vi "xeva-init.vi"() -> (0 "error out":errorcluster, 1 "initialized":bool, 2 "xeva-camref":T2)   [LabVIEW 2015]
uses:
  <vilib>/Xenics Infrared Solutions/Xeneth LabVIEW API/VIs/Controls/Camara.ctl
  <vilib>/Xenics Infrared Solutions/Xeneth LabVIEW API/Xeneth.lvlib
panel:
  in  "settings-file":path=path "D:/Programs/LabView/xenics-xeva-labview/settings/settings-integrationtime15s.xcf"
  in  "calibration-file":path=path "D:/Programs/LabView/xenics-xeva-labview/settings/calibration-170816-15000000us_2795.xca"
  in  "connection-type":T1(ring)=enum."automatic"
  out "status array":bool[](array[boolean])
  # "automatic mode"
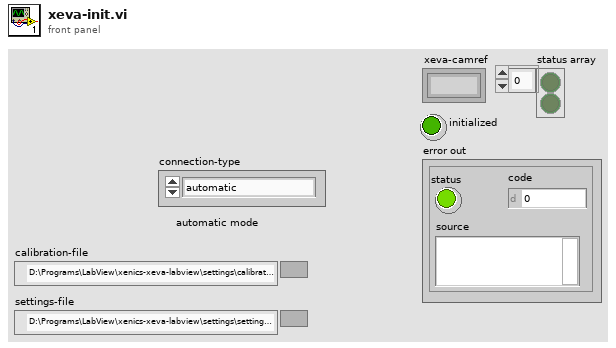
[diagram p1: front panel]
types:
  T1 = enum16{"interactive", "semi-interactive", "automatic"}
  T2 = typedef "Xeneth.lvlib/Camara.ctl" = refnum<k1>
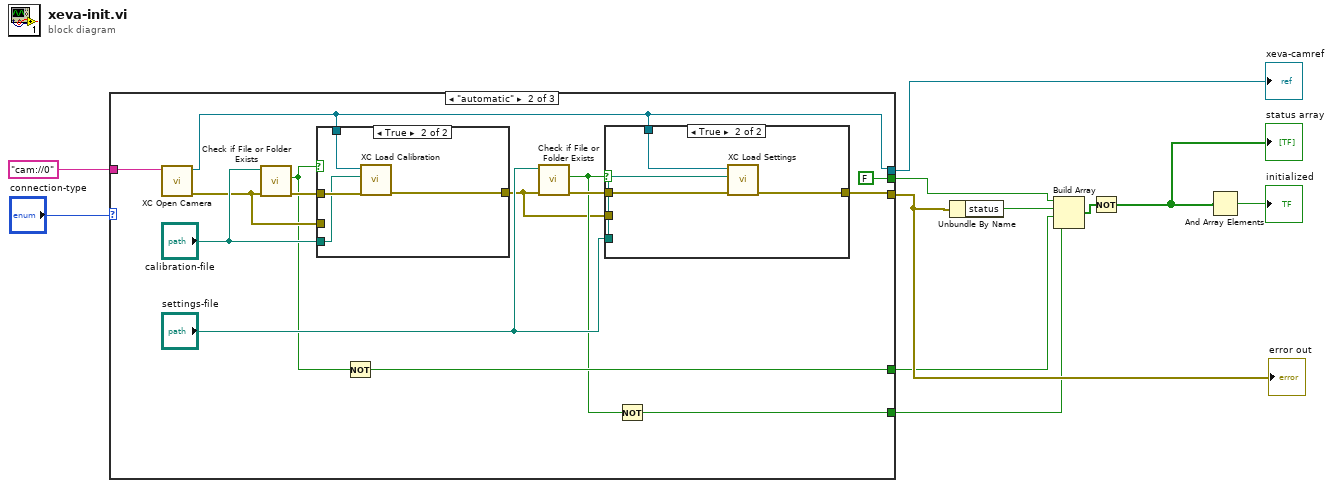
[diagram p0: block diagram]
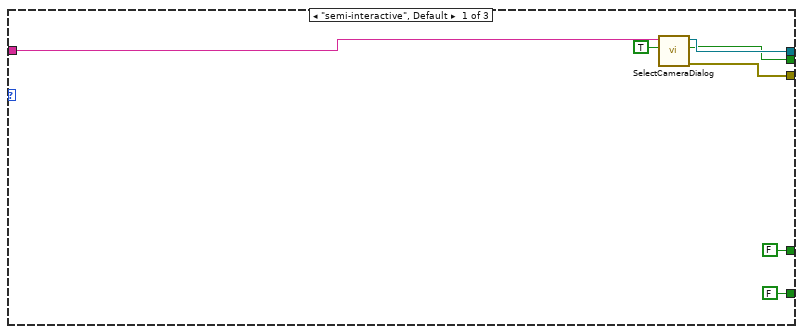
[diagram p2: hidden frame]
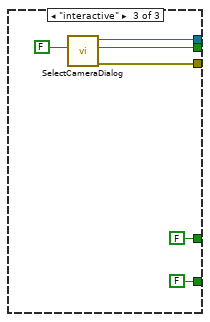
[diagram p5: hidden frame]
diagram:
  n1 = case shown="\"automatic\"" "connection-type" {
    tunnel: [w18 w19 w47] -> w11
    tunnel: [w16 w31 w46] -> w10
    tunnel: [w17 FALSE ("Cancelled") w45] -> w8
    tunnel: "cam://0" ("pCameraName") -> [w15 w32 _]
    tunnel: [FALSE w23 FALSE] -> w2
    tunnel: [FALSE w20 FALSE] -> w1
    frame "semi-interactive", Default {
      n2 = call <vilib>:"SelectCameraDialog.vi"("Direct connct mode (F)"=TRUE, "DefaultConnection"=w15) -> ("error out"=w16:errorcluster, "Cancelled"=w17:bool, "Cam Ref Out"=w18:T2)  [unwired: 7 in]
    }
    frame "automatic" {
      n3 = call <vilib>:"XC Open Camera.vi"("pCameraName"=w32) -> ("error out"=w26:errorcluster, "Cam Ref"=w19:T2)  [unwired: 9 in]
      n4 = call <vilib>:"Check if File or Folder Exists.vi"("error in (no error)"=w26, "path"="calibration-file") -> ("error out"=w27:errorcluster, "file or folder exists?"=w24:bool)  [unwired: 7 in, 1 out]
      n5 = case shown="True" w24 {
        tunnel: w19 -> [_ w42]
        tunnel: w27 -> [_ w41]
        tunnel: [w38 w40] -> w21
        tunnel: "calibration-file" -> [_ w39]
        tunnel: w26 -> [w38 _]
        frame False {
        }
        frame True {
          n6 = call <vilib>:"XC Load Calibration.vi"("error in (no error)"=w41, "p_cFileName"=w39, "Cam Ref"=w42) -> ("error out"=w40:errorcluster)  [unwired: 7 in, 1 out]
        }
      }
      n7 = Not(x=w24) -> (.not. x?=w23:bool)
      n8 = call <vilib>:"Check if File or Folder Exists.vi"("error in (no error)"=w21, "path"="settings-file") -> ("error out"=w25:errorcluster, "file or folder exists?"=w22:bool)  [unwired: 7 in, 1 out]
      n9 = case shown="True" w22 {
        tunnel: w19 -> [_ w37]
        tunnel: w25 -> [_ w36]
        tunnel: [w33 w35] -> w31
        tunnel: "settings-file" -> [_ w34]
        tunnel: w21 -> [w33 _]
        frame False {
        }
        frame True {
          n10 = call <vilib>:"XC Load Settings.vi"("error in (no error)"=w36, "p_cFileName"=w34, "Cam Ref"=w37) -> ("error out"=w35:errorcluster)  [unwired: 7 in, 1 out]
        }
      }
      n11 = Not(x=w22) -> (.not. x?=w20:bool)
    }
    frame "interactive" {
      n12 = call <vilib>:"SelectCameraDialog.vi"("Direct connct mode (F)"=FALSE) -> ("error out"=w46:errorcluster, "Cancelled"=w45:bool, "Cam Ref Out"=w47:T2)  [unwired: 8 in]
    }
  }
  "xeva-camref" <- w11
  "error out" <- w10
  n13 = Unbundle By Name(w10) -> ("status"=w9:bool)
  n14 = Build Array(w8, w9, w2, w1) -> (w7:bool[])
  n15 = Not(x=w7) -> (.not. x?=w5:bool[])
  "status array" <- w5
  n16 = And Array Elements(Boolean array=w5) -> (logical AND=→"initialized":bool)
